vi "Slew Rate.vi"(6 "Initial Output":dbl, 7 "Disable":bool, 8 "error in (no error)":errorcluster, 10 "Units / Second":dbl, 11 "Input":dbl) -> (0 "error out":errorcluster, 2 "Slew Controlled":bool, 3 "Output":dbl)   [LabVIEW 2015]
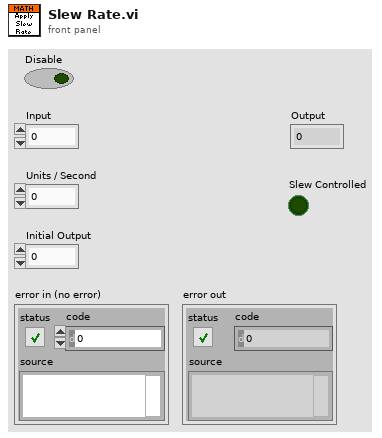
[diagram p1: front panel]
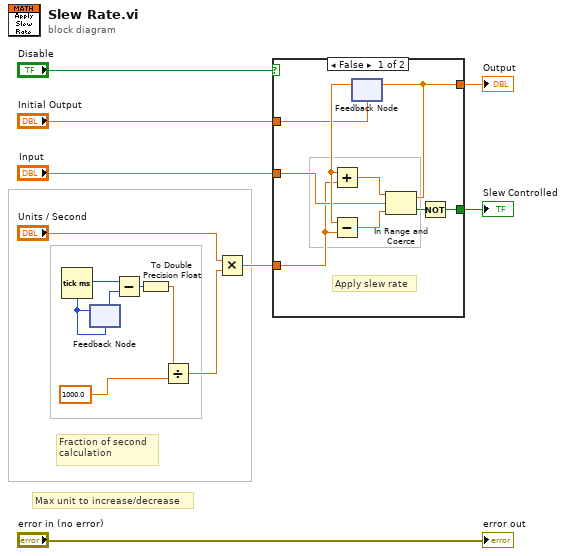
[diagram p0: block diagram]
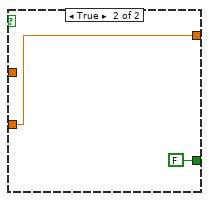
[diagram p2: hidden frame]
diagram:
  # "Max unit to increase/decrease"
  # "Fraction of second\ncalculation"
  n1 = Tick Count (ms)() -> (millisecond timer value=w9:u32)
  n2 = feedback #1(w9) -> (w10:u32)
  n3 = feedback-in #1(w9) -> ()
  n4 = Subtract(x=w9, y=w10) -> (x-y=w8:u32)
  n5 = To Double Precision Float(number=w8) -> (double precision float=w5:dbl)
  n6 = Divide(x=w5, y=1000.0) -> (x/y=w6:dbl)
  n7 = Multiply(x="Units / Second", y=w6) -> (x*y=w3:dbl)
  n8 = case shown="False" "Disable" {
    tunnel: "Input" -> [w20 w25]
    tunnel: [w19 w25] -> w12
    tunnel: w3 -> [w17 _]
    tunnel: "Initial Output" -> [w16 _]
    tunnel: [w15 FALSE] -> w1
    frame False {
      # "Apply slew rate"
      n9 = feedback #2(w16) -> (w23:dbl)
      n10 = Add(x=w23, y=w17) -> (x+y=w21:dbl)
      n11 = Subtract(x=w23, y=w17) -> (x-y=w22:dbl)
      n12 = In Range and Coerce(upper limit=w21, x=w20, lower limit=w22) -> (coerced(x)=w19:dbl, In Range?=w18:bool)
      n13 = feedback-in #2(w19) -> ()
      n14 = Not(x=w18) -> (.not. x?=w15:bool)
    }
    frame True {
    }
  }
  "Output" <- w12
  "Slew Controlled" <- w1
  "error out" <- "error in (no error)"
